vi "CreateErrorProcessor.vi"(7 "elements to preallocate per priority (16)":i32=16, 8 "error in":errorcluster, 9 "default reporting parameter":T1, 10 "reporting parameters":T1[](array[typedef]), 11 "number of priorities":i32=3) -> (0 "error out":errorcluster, 2 "error reporter":refnum<class "ErrorReporter.lvclass">, 3 "error processor":refnum<class "ErrorProcessor.lvclass">)   [LabVIEW 2013, in "CLM_ErrorHandler.lvlib" / "ErrorProcessor.lvclass"]
uses:
  ErrorProcessor.lvclass
  ErrorReporter/ReportingParameter.ctl
  ErrorReporter/ErrorReporter.lvclass
  ErrorProcessor.lvclass/ErrorProcessor.ctl
  <vilib>/CLM/LocalMessenger/PriorityLocalMessage/CLM_PriorityLocalMessage.lvclass
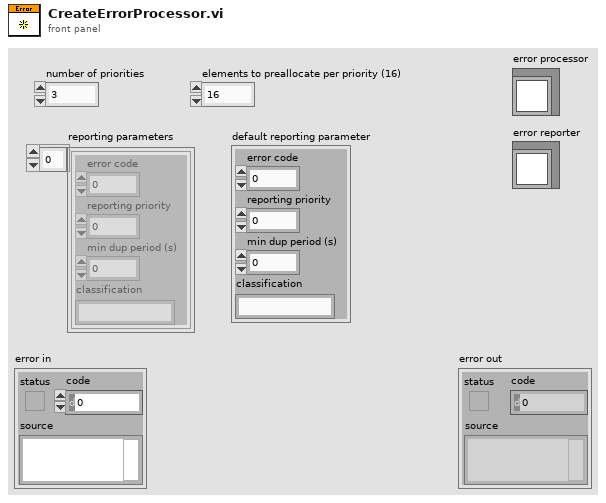
[diagram p1: front panel]
types:
  T1 = typedef "CLM_ErrorHandler.lvlib/ErrorReporter.lvclass/ReportingParameter.ctl" = cluster{"error code":i32, "reporting priority":i32, "min dup period (s)":dbl, "classification":string}
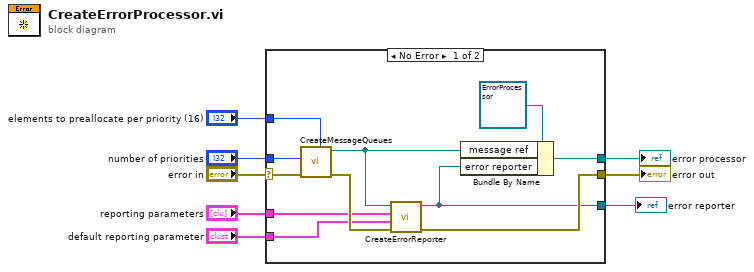
[diagram p0: block diagram]
diagram:
  n1 = case shown="No Error" "error in" {
    selector: "error in" -> [w17 w20]
    tunnel: [w14 w20] -> w7
    tunnel: [w18 _] -> w6
    tunnel: "number of priorities" -> [w13 _]
    tunnel: "elements to preallocate per priority (16)" -> [w12 _]
    tunnel: "reporting parameters" -> [w11 _]
    tunnel: "default reporting parameter" -> [w10 _]
    tunnel: [w9 _] -> w1
    frame No Error {
      n2 = call <vilib>:"CreateMessageQueues.vi"("elements to preallocate per priority (0)"=w12, "error in"=w17, "number of priorities"=w13) -> ("error out"=w15:errorcluster, "message ref out"=w16:refnum<class "CLM_PriorityLocalMessage.lvclass">)  [unwired: 4 in, 3 out]
      n3 = call "CreateErrorReporter.vi"("error in"=w15, "default reporting parameter"=w10, "reporting parameters"=w11, "message ref in"=w16) -> ("error out"=w14:errorcluster, "error reporter out"=w9:refnum<class "ErrorReporter.lvclass">)  [unwired: 6 in]
      n4 = Bundle By Name(cluster=refnum<class "ErrorProcessor.lvclass"> refnum ("CLM_ErrorHandler.lvlib:ErrorProcessor.lvclass"), "message ref"=w16, "error reporter"=w9) -> (w18:refnum<class "ErrorProcessor.lvclass">)
    }
    frame Error {
    }
  }
  "error out" <- w7
  "error processor" <- w6
  "error reporter" <- w1
